vi "Construct Network Sink.vi"(7 "LogLevel":T1, 9 "Local ID":string, 10 "Remote Port":u16, 11 "Remote IP":string) -> (3 "Network Sink out":refnum<class "Network Sink.lvclass">)   [LabVIEW 2017, in "Network Sink.lvlib" / "Network Sink.lvclass"]
uses:
  <vilib>/gpm_packages/@cs/event-logger/Source/Network Sink/Network Sink/Network Sink.lvclass
  C:/Program Files/National Instruments/LabVIEW 2017/vi.lib/gpm_packages/@cs/event-logger/Source/Composed Log/Log Sink/Log Sink.lvclass
  <vilib>/gpm_packages/@cs/event-logger/Source/Composed Log/Types/Log Level.ctl
  <vilib>/gpm_packages/@cs/event-logger/Source/Network Sink/Network Sink/Network Sink.lvclass/Network Sink.ctl
  <vilib>/gpm_packages/@cs/event-logger/Source/Composed Log/Log Sink/Log Sink.lvclass/Log Sink.ctl
  <vilib>/gpm_packages/@cs/event-logger/Source/Composed Log/Log Sink/Log Sink.lvclass
  <vilib>/gpm_packages/@cs/event-logger/Source/Composed Log/Composed Log.lvlib
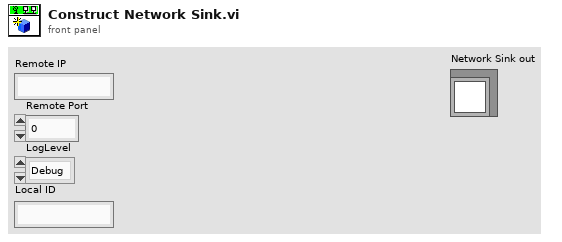
[diagram p1: front panel]
types:
  T1 = typedef "Composed Log.lvlib/Log Level.ctl" = enum16{"Debug", "Info", "Warning", "Error", "Critical"}
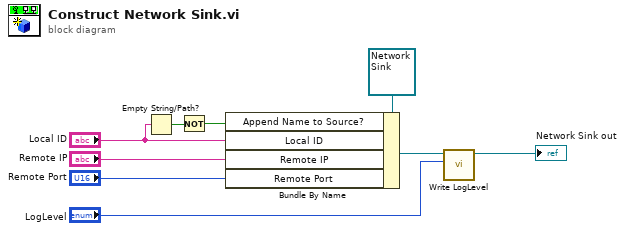
[diagram p0: block diagram]
diagram:
  n1 = Empty String/Path?(string/path="Local ID") -> (empty?=w2:bool)
  n2 = Not(x=w2) -> (.not. x?=w1:bool)
  n3 = Bundle By Name(cluster=refnum<class "Network Sink.lvclass"> refnum ("Network Sink in"), "Append Name to Source?"=w1, "Local ID"="Local ID", "Remote IP"="Remote IP", "Remote Port"="Remote Port") -> (w8:refnum<class "Network Sink.lvclass">)
  n4 = call <vilib>:"Write LogLevel.vi"("LogLevel"="LogLevel", "Log Sink in"=w8) -> ("Log Sink out"=→"Network Sink out":refnum<class "Network Sink.lvclass">)  [unwired: 8 in, 1 out]
